vi "JsonValueToVariant.vi"(8 "error in (no error)":errorcluster, 9 "enums":T1[](array[typedef]), 10 "data type":string, 11 "JSON item":string) -> (0 "error out":errorcluster, 3 "Variant":variant)   [LabVIEW 2018, in "Paser.lvlib"]
uses:
  Paser.lvlib
  Ctrl/Enum.ctl
  Ctrl/EnumValue.ctl
  f5681284-c51d-4f9b-876e-1d86b3bfd3f2.vi
  9524158a-878f-43e4-853c-80c80ecda745.vi
  5ed5c244-1018-4349-a413-a2abb5760e8e.vi
  28f72100-b07b-40fc-a2ba-420b993358cf.vi
  43a21d42-71c0-4cd6-866b-c1729dbe0faa.vi
  4b02d148-bbd0-450f-af8e-831c1d903b5f.vi
  888a06c3-9925-4595-8c84-72e50823d1e5.vi
  d1d49494-9c7d-4a09-85a9-0e0b579641ff.vi
  993a9faa-6b3f-4fc4-b384-c96240fe867a.vi
  <vilib>/JDP Science/JSONtext/JSON text to Variant.vi
  <vilib>/JDP Science/JSONtext/JSONtext.lvlib
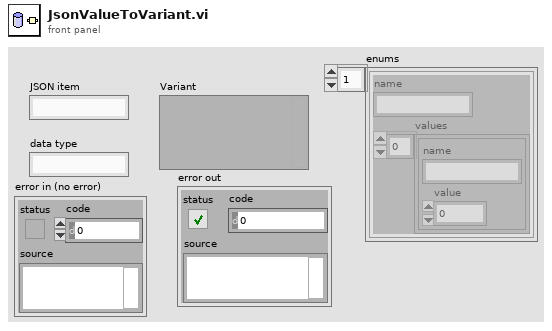
[diagram p1: front panel]
types:
  T1 = typedef "Enum.ctl" = cluster{"name":string, "values":T2[]}
  T2 = typedef "EnumValue.ctl" = cluster{"name":string, "value":i32}
  T3 = typedef "JSONtext.lvlib/JSON Value Type.ctl" = enum16{"Not a JSON Value", "JSON Object", "JSON Array", "String", "Number", "true", "false", "null"}
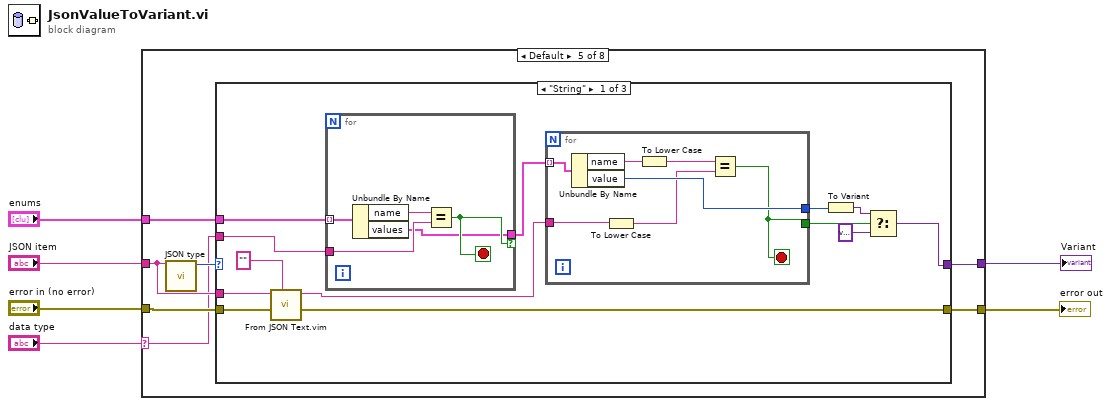
[diagram p0: block diagram]
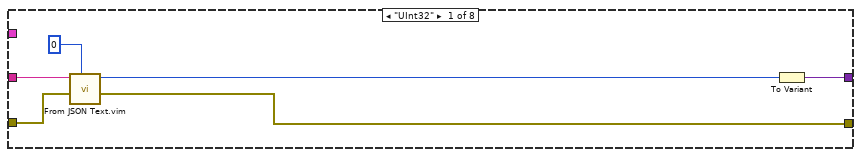
[diagram p2: hidden frame]
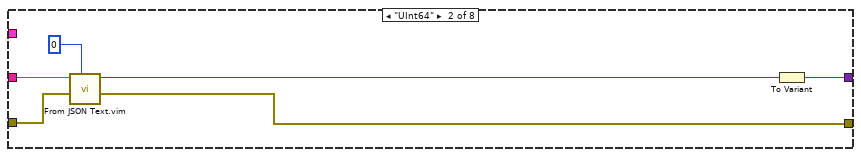
[diagram p3: hidden frame]
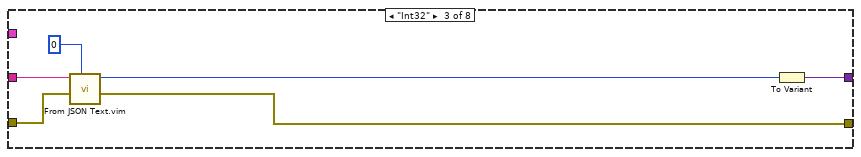
[diagram p4: hidden frame]
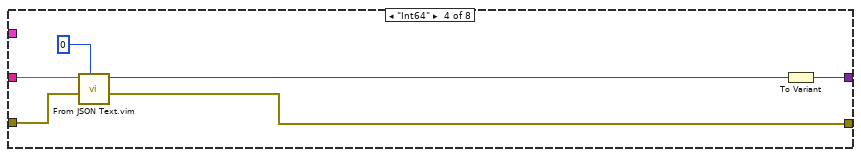
[diagram p5: hidden frame]
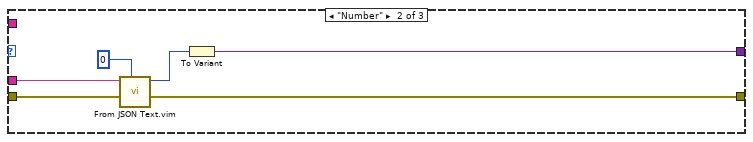
[diagram p6: hidden frame]
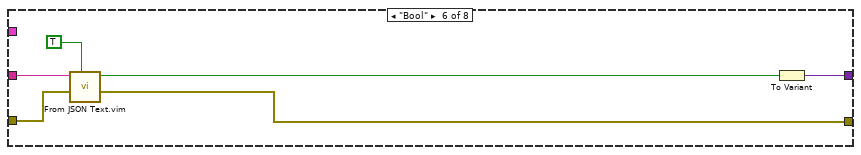
[diagram p8: hidden frame]
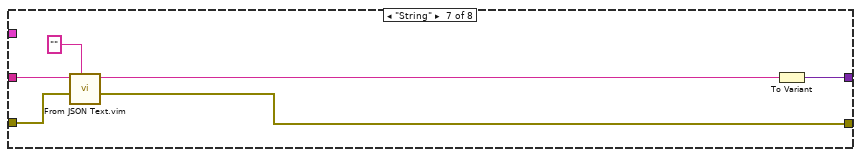
[diagram p9: hidden frame]
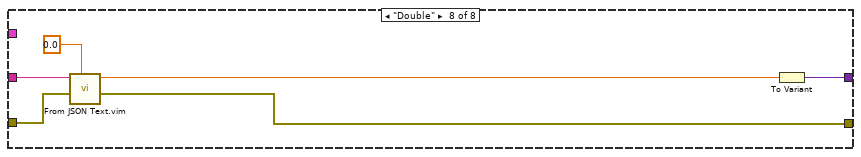
[diagram p10: hidden frame]
diagram:
  n1 = case shown="Default" "data type" {
    selector: "data type" -> [_ _ _ _ w31 _ _ _]
    tunnel: "JSON item" -> [w12 w18 w24 w30 w36 w75 w81 w87]
    tunnel: [w9 w15 w21 w27 w33 w72 w78 w84] -> w6
    tunnel: "error in (no error)" -> [w8 w14 w20 w26 w35 w71 w77 w83]
    tunnel: [w7 w13 w19 w25 w34 w70 w76 w82] -> w2
    tunnel: "enums" -> [_ _ _ _ w32 _ _ _]
    frame "UInt32" {
      n2 = call "From JSON Text.vim"("Data Type and Default Value"=u32 0, "error in (no error)"=w8, "JSON"=w12) -> ("error out"=w7:errorcluster, "Data out"=w10:u32)  [unwired: 7 in]
      n3 = To Variant(anything=w10) -> (Variant=w9:variant)
    }
    frame "UInt64" {
      n4 = call "From JSON Text.vim"("Data Type and Default Value"=u64 0, "error in (no error)"=w14, "JSON"=w18) -> ("error out"=w13:errorcluster, "Data out"=w16:u64)  [unwired: 7 in]
      n5 = To Variant(anything=w16) -> (Variant=w15:variant)
    }
    frame "Int32" {
      n6 = call "From JSON Text.vim"("Data Type and Default Value"=0, "error in (no error)"=w20, "JSON"=w24) -> ("error out"=w19:errorcluster, "Data out"=w22:i32)  [unwired: 7 in]
      n7 = To Variant(anything=w22) -> (Variant=w21:variant)
    }
    frame "Int64" {
      n8 = call "From JSON Text.vim"("Data Type and Default Value"=i64 0, "error in (no error)"=w26, "JSON"=w30) -> ("error out"=w25:errorcluster, "Data out"=w28:i64)  [unwired: 7 in]
      n9 = To Variant(anything=w28) -> (Variant=w27:variant)
    }
    frame Default {
      n10 = call <vilib>:"JSON type.vi"("JSON"=w36) -> ("JSON Value Type"=w37:T3)  [unwired: 9 in, 1 out]
      n11 = case shown="\"String\"" w37 {
        tunnel: w36 -> [w49 w66 _]
        tunnel: w35 -> [w48 w65 w69]
        tunnel: [w47 w64 w69] -> w34
        tunnel: [w38 w63 _] -> w33
        tunnel: w32 -> [w46 _ _]
        tunnel: w31 -> [w45 _ _]
        frame "String" {
          n12 = call "From JSON Text.vim"("Data Type and Default Value"="", "error in (no error)"=w48, "JSON"=w49) -> ("error out"=w47:errorcluster, "Data out"=w43:string)  [unwired: 7 in]
          n13 = for {
            tunnel: w46 -> [w62] mode=indexing
            tunnel: w45 -> [w59]
            tunnel: [w58] -> w44 if=w60
            stop <- w60 stop-if-true
            n14 = Unbundle By Name(w62) -> ("name"=w61:string, "values"=w58:T2[])
            n15 = Equal?(x=w61, y=w59) -> (x = y?=w60:bool)
          }
          n16 = for {
            tunnel: w44 -> [w57] mode=indexing
            tunnel: w43 -> [w52]
            tunnel: [w56] -> w41
            tunnel: [w55] -> w42
            stop <- w55 stop-if-true
            n17 = Unbundle By Name(w57) -> ("name"=w54:string, "value"=w56:i32)
            n18 = To Lower Case(string=w52) -> (all lower case string=w51:string)
            n19 = To Lower Case(string=w54) -> (all lower case string=w53:string)
            n20 = Equal?(x=w53, y=w51) -> (x = y?=w55:bool)
          }
          n21 = To Variant(anything=w41) -> (Variant=w40:variant)
          n22 = Select(t=w40, s=w42, f=variant) -> (s? t:f=w38:variant)
        }
        frame "Number" {
          n23 = call "From JSON Text.vim"("Data Type and Default Value"=0, "error in (no error)"=w65, "JSON"=w66) -> ("error out"=w64:errorcluster, "Data out"=w67:i32)  [unwired: 7 in]
          n24 = To Variant(anything=w67) -> (Variant=w63:variant)
        }
        frame Default {
        }
      }
    }
    frame "Bool" {
      n25 = call "From JSON Text.vim"("Data Type and Default Value"=TRUE, "error in (no error)"=w71, "JSON"=w75) -> ("error out"=w70:errorcluster, "Data out"=w73:bool)  [unwired: 7 in]
      n26 = To Variant(anything=w73) -> (Variant=w72:variant)
    }
    frame "String" {
      n27 = call "From JSON Text.vim"("Data Type and Default Value"="", "error in (no error)"=w77, "JSON"=w81) -> ("error out"=w76:errorcluster, "Data out"=w79:string)  [unwired: 7 in]
      n28 = To Variant(anything=w79) -> (Variant=w78:variant)
    }
    frame "Double" {
      n29 = call "From JSON Text.vim"("Data Type and Default Value"=0.0, "error in (no error)"=w83, "JSON"=w87) -> ("error out"=w82:errorcluster, "Data out"=w85:dbl)  [unwired: 7 in]
      n30 = To Variant(anything=w85) -> (Variant=w84:variant)
    }
  }
  "Variant" <- w6
  "error out" <- w2
